vi "Optimiser - Get New Parameter Values.vi"(7 "Analysis Framework in":refnum<class "Analysis Framework.lvclass">, 8 "error in (no error)":errorcluster, 11 "optimisation cluster":T6) -> (0 "error out":errorcluster, 1 "Parameters":string[][](array[string]), 2 "standard error":string, 3 "standard output":string, 4 "Error":bool, 5 "Optimise Finished":bool)   [LabVIEW 2020, in "CIRCUS_uServices.lvlib" / "Analysis Framework.lvclass"]
uses:
  Analysis Framework.lvclass
  Run Utilities/Optimiser Cell/Optimise parameter - numeric.ctl
  Run Utilities/Optimiser Cell/Optimise parameter - string.ctl
  Run Utilities/Optimiser Cell/Optimiser Results.ctl
  Run Utilities/Optimiser Cell/Name with value pair.ctl
  Run Utilities/Optimiser Cell/Optimisation Strategy.ctl
  Run Utilities/Optimiser Cell/Optimiser Cell.lvclass
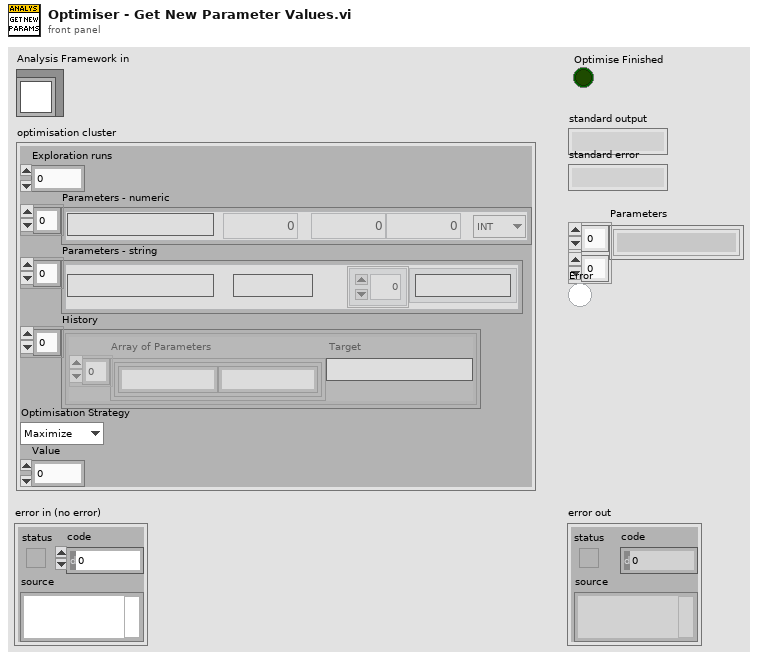
[diagram p1: front panel]
types:
  T1 = typedef "CIRCUS_uServices.lvlib/Run Utilities.lvlib/Optimiser Cell.lvclass/Optimise parameter - numeric.ctl" = cluster{"Name":string, "Start value":dbl, "From":dbl, "To":dbl, "dtype":enum16{"INT", "DBL"}}
  T2 = typedef "CIRCUS_uServices.lvlib/Run Utilities.lvlib/Optimiser Cell.lvclass/Optimise parameter - string.ctl" = cluster{"Name":string, "Start value":string, "Options":string[]}
  T3 = typedef "CIRCUS_uServices.lvlib/Run Utilities.lvlib/Optimiser Cell.lvclass/Optimiser Results.ctl" = cluster{"Array of Parameters":T4[], "Target":string}
  T4 = typedef "CIRCUS_uServices.lvlib/Analysis Framework.lvclass/Name with value pair.ctl" = cluster{"Name":string, "Value":string}
  T5 = typedef "CIRCUS_uServices.lvlib/Run Utilities.lvlib/Optimiser Cell.lvclass/Optimisation Strategy.ctl" = enum16{"Maximize", "Minimize", "Value"}
  T6 = cluster{"Exploration runs":i32, "Parameters - numeric":T1[], "Parameters - string":T2[], "History":T3[], "Optimisation Strategy":T5, "Value":dbl}
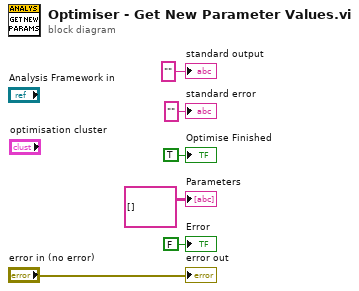
[diagram p0: block diagram]
diagram:
  "error out" <- "error in (no error)"
  "standard output" <- "" ("standard output")
  "standard error" <- "" ("standard error")
  "Optimise Finished" <- TRUE ("Optimise Finished")
  "Parameters" <- string[][] [] ("Targets")
  "Error" <- FALSE ("Error")
